vi "imgread.vi"(9 "error in (no error)":errorcluster, 10 "File Path":path, 11 "Image 2":T1) -> (1 "error out":errorcluster, 2 "Image":T1(plugin-control))   [LabVIEW 2014]
uses:
  <vilib>/vision/Image Controls.llb/IMAQ Image.ctl
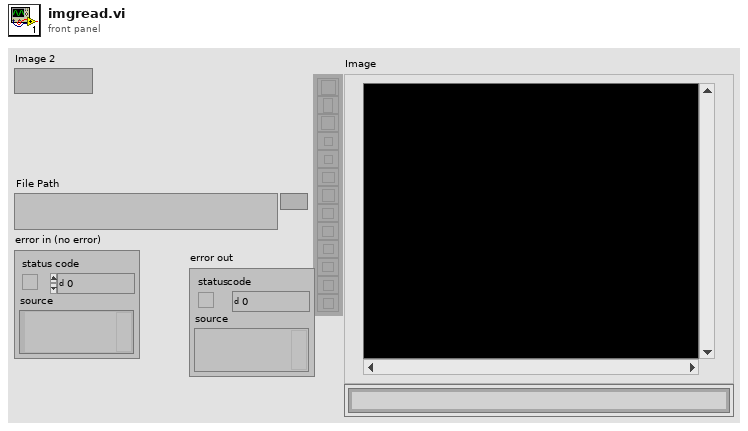
[diagram p1: front panel]
types:
  T1 = typedef "IMAQ Image.ctl" = refnum<image>
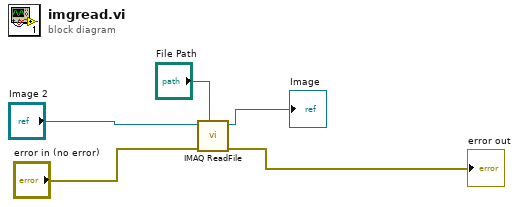
[diagram p0: block diagram]
diagram:
  n1 = call "IMAQ ReadFile"("File Path"="File Path", "error in (no error)"="error in (no error)", "Image"="Image 2") -> ("error out"=→"error out":errorcluster, "Image Out"=→"Image":T1)  [unwired: 4 in, 3 out]
